vi "Bernards_2_2400.vi"() -> ()   [LabVIEW 2018]
uses:
  <vilib>/Utility/file.llb/Write Delimited Spreadsheet (string).vi
  <instrlib>/Keithley 24XX/Public/Data/Read (Single Point).vi
  <instrlib>/Keithley 24XX/Keithley 24XX.lvlib
  <vilib>/Analysis/NI_AALBase.lvlib
panel:
  out "Current (A) 2":dbl format="%.2e"
  out "error 8":string
  in  "Keithley 2401 (new)\nVISA resource #2 = 22":refnum<visa-resource-name>="GPIB0::22::INSTR"
  in  "Delay Gate (s) 2":dbl=60.0 format="%#.3g"
  in  "source/measure (V/I:0)":u16(ring)=1 items=["voltage/current", "current/voltage"]
  in  "Setpoint Array":dbl[](array[numeric])=[-2e-08, -5e-08, -1e-07]
  in  "Measurement Speed (1 PLC)":dbl=1.0 format="%.2g"
  in  "Initial Gate Setting":dbl format="%#.3e"
  in  "Voltage Compliance Limit 2401 (V)":dbl=-0.95 format="%#.3f"
  in  "Current Compliance\nLimit 2401 (A)":dbl=0.10000000009313226
  in  "Delay Gate (s)":dbl=30.0 format="%#.3g"
  in  "Keithley 237 GPIB address":string="17"
  in  "Wait Time Btwn Keithley Readings (ms)":i32=30
  out "Time Btwn Iterations (ms)":i32
  out "Total Elapsed Time (ms)":i32
  out "# Avgs":i32
  out "Current (A)":dbl format="%.2e"
  in  "Total Measure Time (s)":dbl=120.0 format="%#.3g"
  in  "Drain Bias (V)":dbl=-0.6 format="%#.3g"
  in  "Current Compliance\nLimit (A)":dbl=0.5 format="%#.3e"
  in  "Keithley 2400 (old)\nVISA resource #1 = 24":refnum<visa-resource-name>="GPIB0::24::INSTR"
  in  "ApproximateTime Step (ms)":dbl=300.0 format="%#.3g"
  in  "Current Offset":dbl format="%^#_3e"
  out "I-t Measurement\nBy M. Ziffer 7/3/2014":cluster{dbl[], dbl[]}(graph)={[-2.0, -1.95, -1.9, -1.85, -1.8, -1.75, -1.7, -1.65, -1.6, -1.55, -1.5, -1.45, -1.4, -1.35, -1.2999999999999998, -1.25, -1.2, -1.15, -1.1, -1.0499999999999998, -1.0, -0.95, -0.8999999999999999, -0.8499999999999999, -0.7999999999999998, -0.75, -0.7, -0.6499999999999999, -0.5999999999999999, -0.5499999999999998, -0.5, -0.44999999999999996, -0.3999999999999999, -0.34999999999999987, -0.2999999999999998, -0.25, -0.19999999999999996, -0.1499999999999999, -0.09999999999999987, -0.04999999999999982, 0.0, 0.050000000000000266, 0.10000000000000009, 0.1499999999999999, 0.20000000000000018, 0.25, 0.30000000000000027, 0.3500000000000001, 0.40000000000000036, 0.4500000000000002, 0.5, 0.5500000000000003, 0.6000000000000001, 0.6500000000000004, 0.7000000000000002, 0.75, 0.8000000000000003, 0.8500000000000001, 0.9000000000000004, 0.9500000000000002, 1.0, 1.0500000000000003, 1.1, 1.1500000000000004, 1.2000000000000002, 1.25, 1.3000000000000003, 1.35, 1.4000000000000004, 1.4500000000000002, 1.5, 1.5500000000000003, 1.6, 1.6500000000000004, 1.7000000000000002, 1.75, 1.8000000000000003, 1.85, 1.9000000000000004, 1.9500000000000002, 2.0, 1.95, 1.9, 1.85, 1.8, 1.75, 1.7, 1.65, 1.6, 1.55, 1.5, 1.45, 1.4, 1.35, 1.2999999999999998, 1.25, 1.2, 1.15, 1.1, 1.0499999999999998, 1.0, 0.95, 0.8999999999999999, 0.8499999999999999, 0.7999999999999998, 0.75, 0.7, 0.6499999999999999, 0.5999999999999999, 0.5499999999999998, 0.5, 0.44999999999999996, 0.3999999999999999, 0.34999999999999987, 0.2999999999999998, 0.25, 0.19999999999999996, 0.1499999999999999, 0.09999999999999987, 0.04999999999999982, 0.0, -0.050000000000000266, -0.10000000000000009, -0.1499999999999999, -0.20000000000000018, -0.25, -0.30000000000000027, -0.3500000000000001, -0.40000000000000036, -0.4500000000000002, -0.5, -0.5500000000000003, -0.6000000000000001, -0.6500000000000004, -0.7000000000000002, -0.75, -0.8000000000000003, -0.8500000000000001, -0.9000000000000004, -0.9500000000000002, -1.0, -1.0500000000000003, -1.1, -1.1500000000000004, -1.2000000000000002, -1.25, -1.3000000000000003, -1.35, -1.4000000000000004, -1.4500000000000002, -1.5, -1.5500000000000003, -1.6, -1.6500000000000004, -1.7000000000000002, -1.75, -1.8000000000000003, -1.85, -1.9000000000000004, -1.9500000000000002, -2.0], [-0.9617289445307117, -0.9618513744908972, -0.9601574911889584, -0.9603488957746004, -0.9598860982876659, -0.9595594700613103, -0.9590290885663679, -0.9586886097902229, -0.9580144940757807, -0.9570474587019399, -0.9571418538143588, -0.9562287187728303, -0.9551771894828052, -0.9535572870291384, -0.9535421571112963, -0.9533114258642045, -0.9520938012261039, -0.9513117179729429, -0.9508812384355169, -0.9504840780921618, -0.9504173840793213, -0.9482281628421478, -0.9464640811713977, -0.9453356785488072, -0.9439408336230415, -0.9428695575652444, -0.9416178906119992, -0.9396031084275935, -0.9378375248899987, -0.9354517815949719, -0.9324159524550173, -0.928767917889437, -0.9245502864168607, -0.9203528467096396, -0.9146985405384399, -0.908595454304189, -0.9012966039381313, -0.8917361646028689, -0.8808115851751085, -0.8684870433493713, -0.853007079283089, -0.8360736418594031, -0.8154860511533626, -0.7920970894092216, -0.7641180332150388, -0.7294003786125389, -0.6854183749419586, -0.6263231964633708, -0.5399961516707377, -0.4044042921440459, -0.19129744134883978, 0.11936942255465804, 0.5420583260977958, 1.0996962734707192, 1.8318907919106253, 2.7834859177196174, 3.9948214605959804, 5.494887344369723, 7.293988211209965, 9.39251059714275, 11.765998658717283, 14.371720946722268, 17.153138293174568, 20.070768287470067, 23.082285540692517, 26.15604905590766, 29.26009131920428, 32.38734131897913, 35.54092126952808, 38.70923397757575, 41.89103456238207, 45.09512285116253, 48.318234786641504, 51.57411300669423, 54.84161623237131, 58.130390342544004, 61.4596508891188, 64.79419021952893, 68.17503711098149, 71.57587551887687, 75.0023346626475, 71.8977923333163, 68.72637799211101, 65.51757272894447, 62.2950059155054, 59.076872390492845, 55.84672949319313, 52.615591470047114, 49.383497814590335, 46.15858586388574, 42.93308596012382, 39.714879010509975, 36.494540522470736, 33.276879251143754, 30.087779593472593, 26.903443634933772, 23.758388169345494, 20.669969771208738, 17.671195580039395, 14.804861569698371, 12.12778391916459, 9.68736655227705, 7.528128139792144, 5.673530623057721, 4.128839936603901, 2.8787577310032053, 1.895544581260216, 1.1383875896205915, 0.5622048852612092, 0.12746496878202787, -0.18928305409978952, -0.4042961076690051, -0.5411369085387429, -0.6286316214282486, -0.6871327837574404, -0.7298882072135505, -0.7640718647157413, -0.7921132761963248, -0.8155779431543743, -0.8358809022810104, -0.8523300154596555, -0.8668520109778625, -0.8802307520791266, -0.8907705198464766, -0.8998007445608903, -0.9078572589377096, -0.9150023626386364, -0.9215738644543149, -0.925261336930741, -0.9288795566582202, -0.9332418679701618, -0.9352489739462505, -0.9376688708058178, -0.9394550911063516, -0.9405290371496502, -0.9430050037047499, -0.9440335043698243, -0.9453382929096107, -0.9473152502994113, -0.9474565926568992, -0.9494901203645137, -0.94896546821346, -0.9503187058651598, -0.9511280452203158, -0.9523093469306558, -0.9532668704811476, -0.9541692143312739, -0.9545545822386634, -0.955485183435348, -0.9561708134622656, -0.956805602515258, -0.9577699122788996, -0.9578049002139094, -0.9580356870856992, -0.958780001168953, -0.9592832934359943, -0.9588639388381576, -0.959203916992021, -0.9603773199952523, -0.9611007191920772, -0.9623172869609168]}
  in  "First bias settle (ms)":dbl=2000.0 format="%#.2f"
  out "Outputfile":path
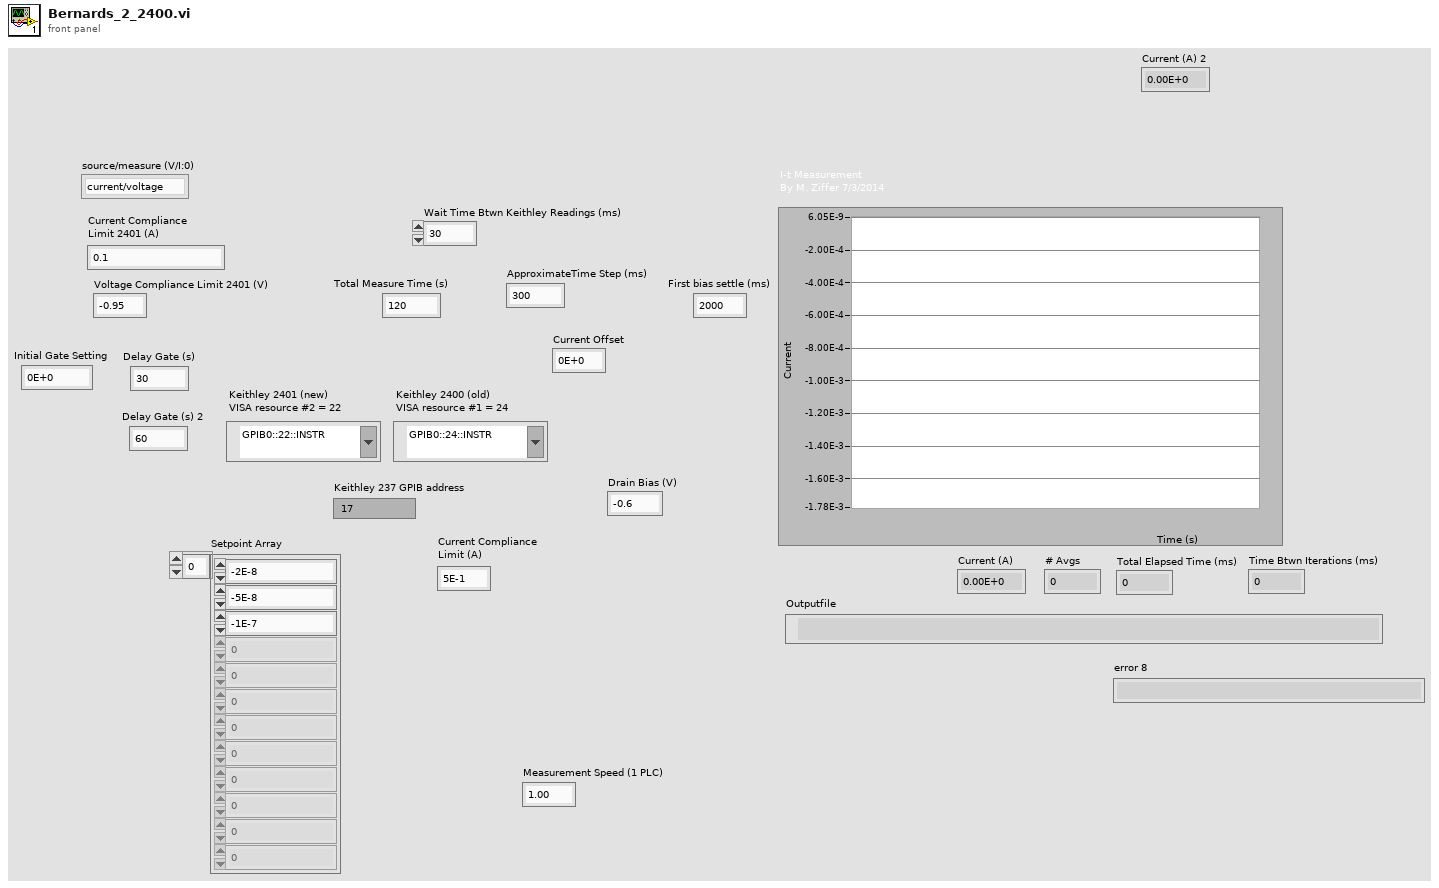
[diagram p1: front panel]
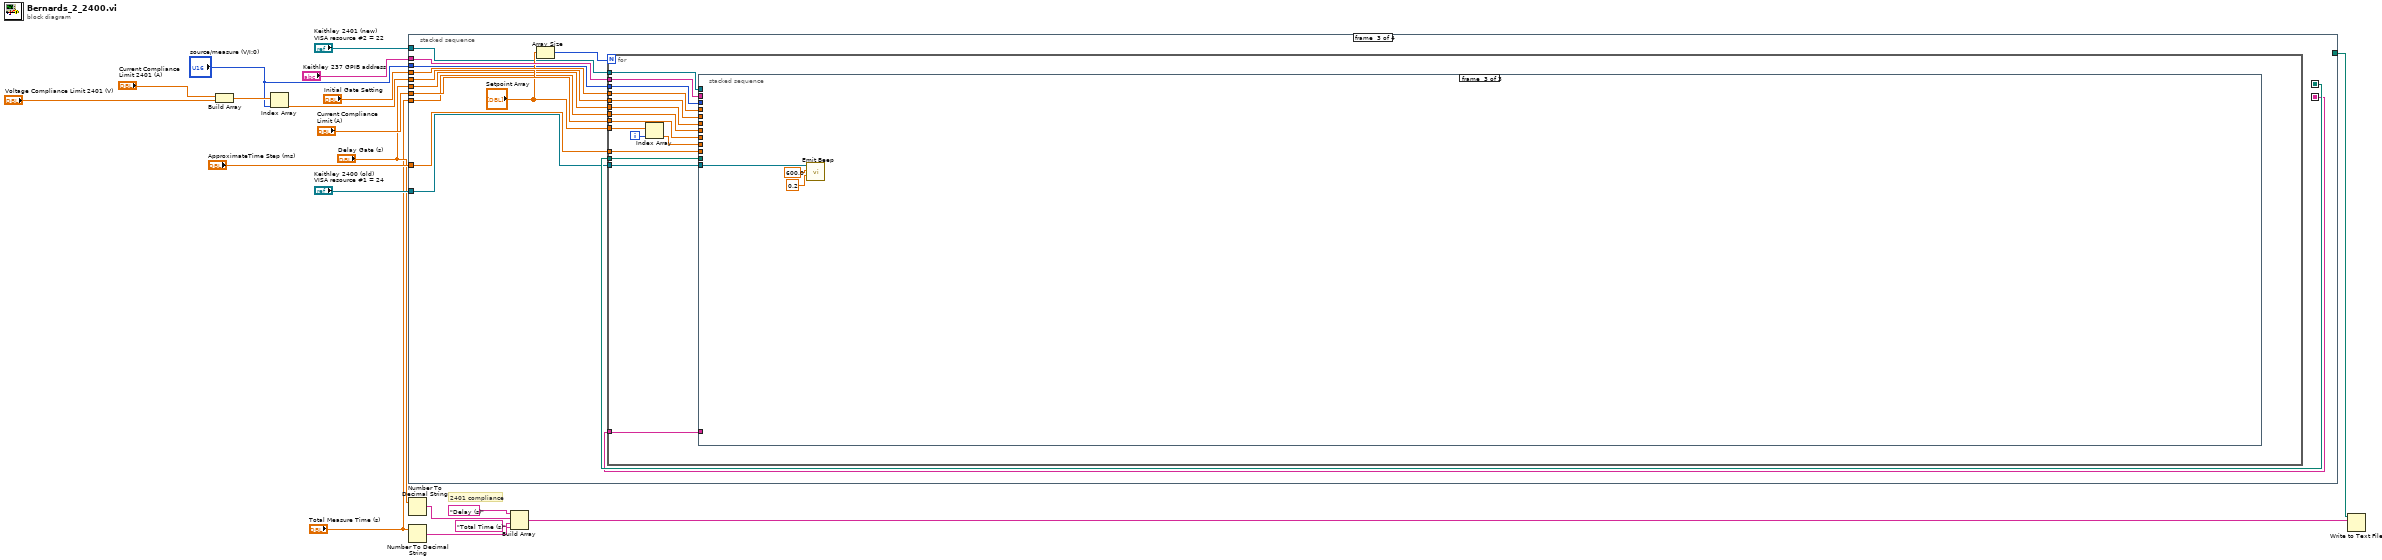
[diagram p0: block diagram]
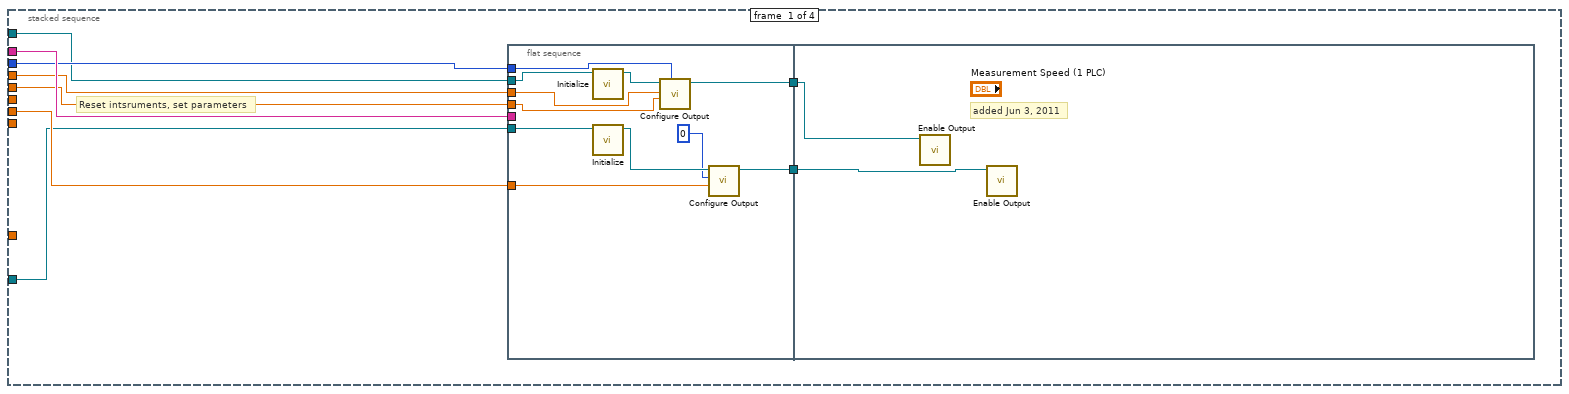
[diagram p2: hidden frame]
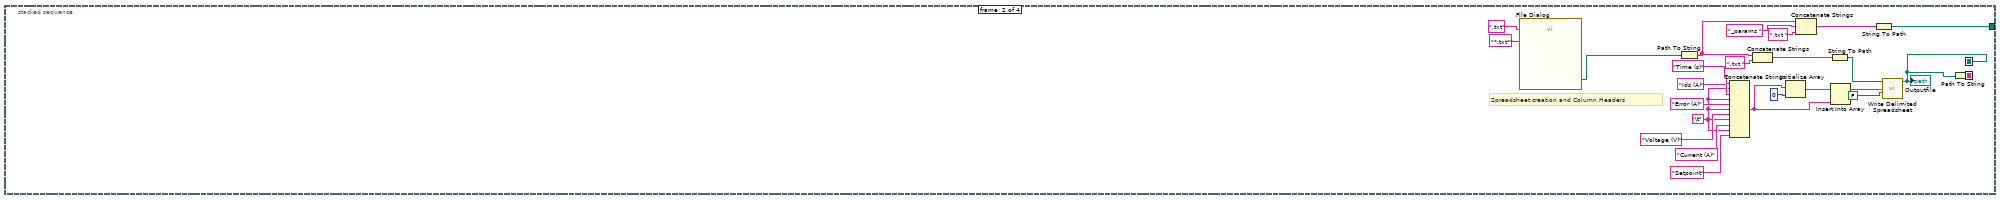
[diagram p3: hidden frame]
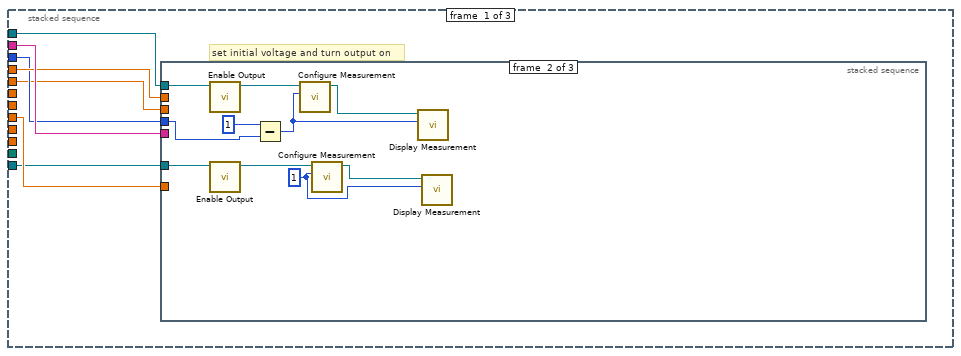
[diagram p4: hidden frame]
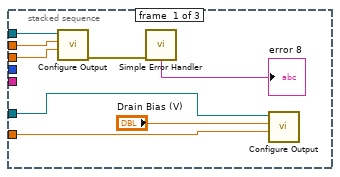
[diagram p5: hidden frame]
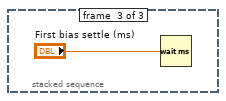
[diagram p6: hidden frame]
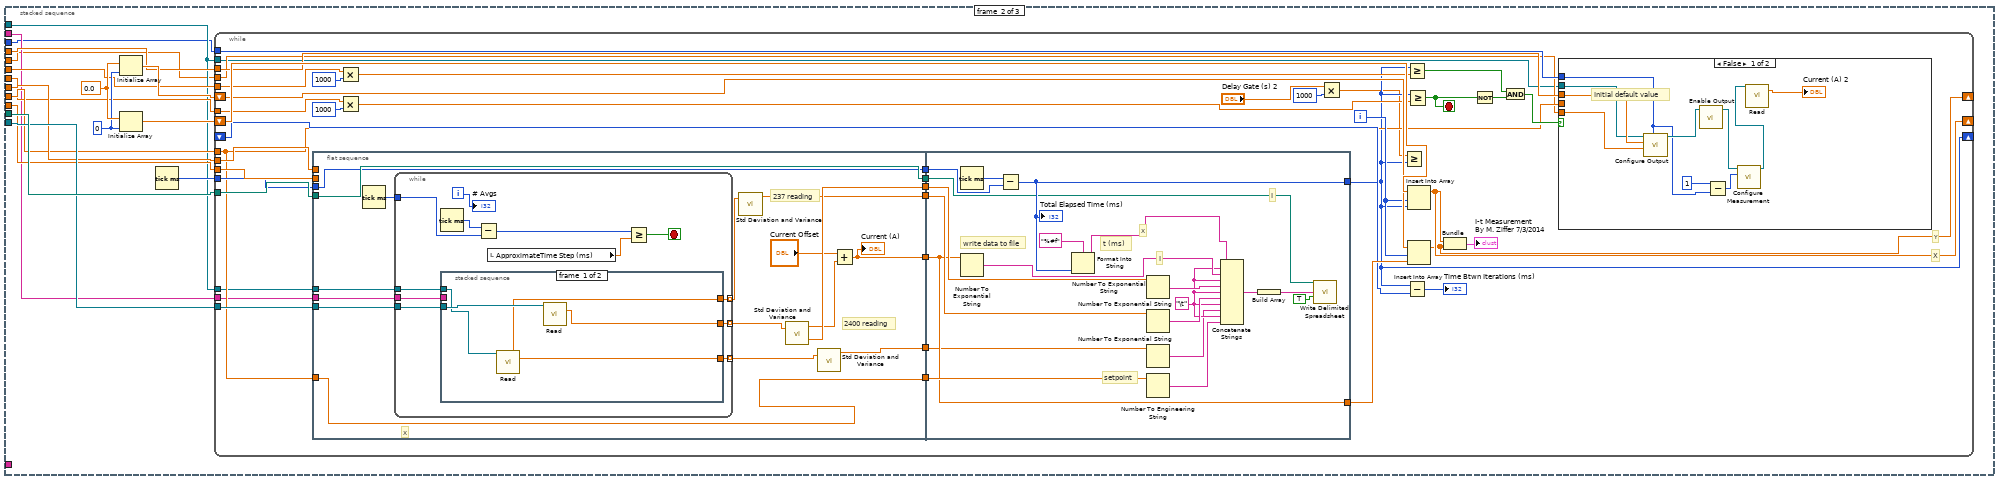
[diagram p7: hidden frame]
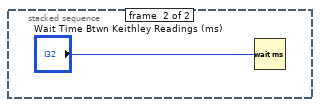
[diagram p8: hidden frame]
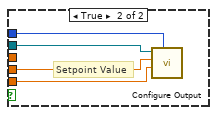
[diagram p9: hidden frame]
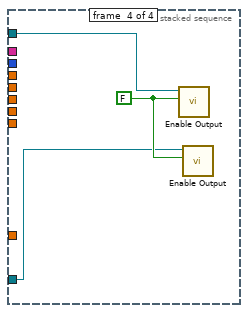
[diagram p10: hidden frame]
diagram:
  # "2401 compliance"
  n1 = Build Array("Current Compliance\nLimit 2401 (A)", "Voltage Compliance Limit 2401 (V)") -> (w4:dbl[])
  n2 = Index Array(array=w4, index="source/measure (V/I:0)") -> (element=w2:dbl)
  n3 = stacked-sequence {
    seq-local: [_ w47 _ _] -> [_ _ w79 _]
    seq-local: [_ w66 _ _] -> [_ _ w78 _]
    tunnel: "ApproximateTime Step (ms)" -> [_ _ w80 _]
    tunnel: "Keithley 2400 (old)\nVISA resource #1 = 24" -> [w27 _ w76 w252]
    tunnel: "Current Compliance\nLimit (A)" -> [w28 _ w77 _]
    tunnel: "Keithley 237 GPIB address" -> [w26 _ w74 _]
    tunnel: "Initial Gate Setting" -> [w22 _ w75 _]
    tunnel: "source/measure (V/I:0)" -> [w25 _ w68 _]
    tunnel: [_ w42 _ _] -> w13
    tunnel: "Delay Gate (s)" -> [_ _ w71 _]
    tunnel: "Total Measure Time (s)" -> [_ _ w70 _]
    tunnel: "Keithley 2401 (new)\nVISA resource #2 = 22" -> [w24 _ w69 w253]
    tunnel: w2 -> [w23 _ w67 _]
    frame #0 {
      # "Reset intsruments, set parameters"
      n4 = flat-sequence {
        tunnel: w27 -> [w38]
        tunnel: w28 -> [w34]
        tunnel: w26 -> [_]
        tunnel: w25 -> [w33]
        tunnel: w24 -> [w36]
        tunnel: w23 -> [w32]
        tunnel: w22 -> [w31]
        tunnel: [w39] -> w21
        tunnel: [w29] -> w20
        tunnel: w21 -> [w41]
        tunnel: w20 -> [w40]
        frame #0 {
          n5 = call <instrlib>:"Initialize.vi"("VISA resource name"=w36) -> ("VISA resource name out"=w35:refnum<visa-resource-name>)  [unwired: 9 in, 1 out]
          n6 = call <instrlib>:"Initialize.vi"("VISA resource name"=w38) -> ("VISA resource name out"=w37:refnum<visa-resource-name>)  [unwired: 9 in, 1 out]
          n7 = call <instrlib>:"Configure Output.vi"("Source Mode  (0: Voltage)"=w33, "Compliance  Level (0.1)"=w32, "Output Level (0)"=w31, "VISA resource name"=w35) -> ("VISA resource name out"=w29:refnum<visa-resource-name>)  [unwired: 2 in, 5 out]
          n8 = call <instrlib>:"Configure Output.vi"("Compliance  Level (0.1)"=w34, "Output Level (0)"=0, "VISA resource name"=w37) -> ("VISA resource name out"=w39:refnum<visa-resource-name>)  [unwired: 3 in, 5 out]
        }
        frame #1 {
          # "added Jun 3, 2011"
          n9 = call <instrlib>:"Enable Output.vi"("VISA resource name"=w40) -> ()  [unwired: 2 in, 9 out]
          n10 = call <instrlib>:"Enable Output.vi"("VISA resource name"=w41) -> ()  [unwired: 2 in, 9 out]
        }
      }
    }
    frame #1 {
      w49 = "\t"
      # "Spreadsheet creation and Column Headers"
      n11 = call "File Dialog"("default name"=".txt", "pattern (all files)"="*.txt*") -> ("selected path"=w53:path)  [unwired: 5 in, 8 out]
      n12 = Path To String(path=w53) -> (string=w44:string)
      n13 = Concatenate Strings("Time (s)", w49, "Ids (A)", w49, "Error (A)", w49, "Voltage (V)", w49, "Current (A)", w49, "Setpoint") -> (w64:string)
      n14 = Concatenate Strings(w44, ".txt " ("string")) -> (w52:string)
      n15 = Initialize Array(w64, 0 ("dimension size")) -> (w63:string[])
      n16 = Concatenate Strings(w44, "_params " ("string"), ".txt " ("string")) -> (w43:string)
      n17 = String To Path(string=w52) -> (path=w51:path)
      n18 = Insert Into Array(array=w63, new element=w64) -> (w56:string[])  [unwired: 1 in]
      n19 = String To Path(string=w43) -> (path=w42:path)
      n20 = call-poly <vilib>:"Write Delimited Spreadsheet.vi"("file path (dialog if empty)"=w51, "1D data"=w56, "append to file? (new file:F)"=FALSE) -> ("new file path (Not A Path if cancelled)"=w47:path)  [unwired: 11 in, 1 out]
      "Outputfile" <- w47
      n21 = Path To String(path=w47) -> (string=w66:string)
    }
    frame #2 {
      n22 = Array Size(array="Setpoint Array") -> (size(s)=w72:i32)
      n23 = for {
        N: w72 -> [_]
        tunnel: w80 -> [w95]
        tunnel: w79 -> [w94]
        tunnel: w78 -> [w93]
        tunnel: w77 -> [w92]
        tunnel: w76 -> [w91]
        tunnel: w75 -> [w90]
        tunnel: w74 -> [w84]
        tunnel: "Setpoint Array" -> [w89]
        tunnel: w71 -> [w86]
        tunnel: w70 -> [w85]
        tunnel: w69 -> [w83]
        tunnel: w68 -> [w82]
        tunnel: w67 -> [w81]
        i -> [w87]
        n24 = Index Array(array=w89, index=w87) -> (element=w88:dbl)
        n25 = stacked-sequence {
          tunnel: w95 -> [_ w131 _]
          tunnel: w94 -> [_ w138 _]
          tunnel: w93 -> [_ _ _]
          tunnel: w92 -> [w102 w132 _]
          tunnel: w91 -> [w101 w133 w251]
          tunnel: w90 -> [w98 w129 _]
          tunnel: w84 -> [w100 w125 _]
          tunnel: w88 -> [_ w128 _]
          tunnel: w86 -> [_ w127 _]
          tunnel: w85 -> [_ w126 _]
          tunnel: w83 -> [w99 w124 _]
          tunnel: w82 -> [w97 w123 _]
          tunnel: w81 -> [w96 w122 _]
          frame #0 {
            # "set initial voltage and turn output on"
            n26 = stacked-sequence {
              tunnel: w101 -> [w109 w120 _]
              tunnel: w102 -> [w110 _ _]
              tunnel: w100 -> [_ _ _]
              tunnel: w99 -> [w107 w119 _]
              tunnel: w98 -> [w106 _ _]
              tunnel: w97 -> [_ w115 _]
              tunnel: w96 -> [w105 _ _]
              frame #0 {
                n27 = call <instrlib>:"Configure Output.vi"("Compliance  Level (0.1)"=w105, "Output Level (0)"=w106, "VISA resource name"=w107) -> ("error out"=w104:errorcluster)  [unwired: 3 in, 5 out]
                n28 = call <vilib>:"Simple Error Handler.vi"("error in (no error)"=w104) -> ("message"=→"error 8":string)  [unwired: 1 in, 7 out]
                n29 = call <instrlib>:"Configure Output.vi"("Compliance  Level (0.1)"=w110, "Output Level (0)"="Drain Bias (V)", "VISA resource name"=w109) -> ()  [unwired: 3 in, 6 out]
              }
              frame #1 {
                w111 = 1
                n30 = call <instrlib>:"Enable Output.vi"("VISA resource name"=w119) -> ("VISA resource name out"=w118:refnum<visa-resource-name>)  [unwired: 2 in, 8 out]
                n31 = call <instrlib>:"Enable Output.vi"("VISA resource name"=w120) -> ("VISA resource name out"=w117:refnum<visa-resource-name>)  [unwired: 2 in, 8 out]
                n32 = Subtract(x=1, y=w115) -> (x-y=w112:i32)
                n33 = call <instrlib>:"Configure Measurement.vi"("Function (0: Volts)"=w112, "VISA resource name"=w118) -> ("VISA resource name out"=w113:refnum<visa-resource-name>)  [unwired: 8 in, 1 out]
                n34 = call <instrlib>:"Configure Measurement.vi"("Function (0: Volts)"=w111, "VISA resource name"=w117) -> ("VISA resource name out"=w114:refnum<visa-resource-name>)  [unwired: 8 in, 1 out]
                n35 = call <instrlib>:"Display Measurement.vi"("Displayed Measurement (0: Voltage)"=w112, "VISA resource name"=w113) -> ()  [unwired: 8 in, 2 out]
                n36 = call <instrlib>:"Display Measurement.vi"("Displayed Measurement (0: Voltage)"=w111, "VISA resource name"=w114) -> ()  [unwired: 8 in, 2 out]
              }
              frame #2 {
                n37 = Wait (ms)(milliseconds to wait="First bias settle (ms)") -> ()  [unwired: 1 out]
              }
            }
          }
          frame #1 {
            w134 = 0
            w135 = 0.0
            n38 = Initialize Array(w135, w134) -> (w136:dbl[])
            n39 = Initialize Array(w135, w134) -> (w137:dbl[])
            n40 = Tick Count (ms)() -> (millisecond timer value=w130:u32)
            n41 = while {
              shift-left: w136 -> [w177]
              shift-right: [w172] -> _
              shift-left: w137 -> [w178]
              shift-right: [w174] -> _
              tunnel: w138 -> [w179]
              tunnel: w133 -> [w176]
              tunnel: w132 -> [w175]
              tunnel: w131 -> [w170]
              tunnel: w130 -> [w165]
              shift-right: [w147] -> _
              shift-left: _ -> [w169]
              tunnel: w125 -> [w156]
              tunnel: w129 -> [w162]
              tunnel: w128 -> [w157]
              tunnel: w127 -> [w144]
              tunnel: w126 -> [w143]
              tunnel: w124 -> [w142]
              tunnel: w124 -> [w139]
              tunnel: w123 -> [w141]
              tunnel: w122 -> [w140]
              i -> [w171]
              stop <- w161 stop-if-true
              # "X"
              # "X"
              # "Y"
              n42 = flat-sequence {
                tunnel: w179 -> [w190]
                tunnel: [w190] -> w155
                tunnel: w176 -> [w184]
                tunnel: w175 -> [_]
                tunnel: w170 -> [_]
                tunnel: w165 -> [w189]
                tunnel: [w189] -> w154
                tunnel: w157 -> [w188]
                tunnel: [w188] -> w153
                tunnel: w156 -> [w191]
                tunnel: [w196] -> w152
                tunnel: [w192] -> w151
                tunnel: [w187] -> w150
                tunnel: [w186] -> w145
                tunnel: w142 -> [w185]
                tunnel: [w220] -> w173
                tunnel: w155 -> [w215]
                tunnel: w154 -> [w227]
                tunnel: [w226] -> w147
                tunnel: w153 -> [w223]
                tunnel: w152 -> [w229]
                tunnel: w151 -> [w220]
                tunnel: w150 -> [w222]
                tunnel: w145 -> [w216]
                frame #0 {
                  # "2400 reading"
                  # "237 reading"
                  n43 = Tick Count (ms)() -> (millisecond timer value=w193:u32)
                  n44 = while {
                    tunnel: w193 -> [w207]
                    tunnel: w191 -> [w202]
                    tunnel: w185 -> [w201]
                    tunnel: w184 -> [w200]
                    tunnel: [w199] -> w183 mode=indexing
                    tunnel: [w198] -> w182 mode=indexing
                    tunnel: [w197] -> w181 mode=indexing
                    i -> [w208]
                    stop <- w205 stop-if-true
                    n45 = Tick Count (ms)() -> (millisecond timer value=w204:u32)
                    n46 = stacked-sequence {
                      tunnel: w202 -> [_ _]
                      tunnel: w201 -> [w212 _]
                      tunnel: w200 -> [w213 _]
                      tunnel: [w211 _] -> w199
                      tunnel: [w210 _] -> w198
                      tunnel: [w209 _] -> w197
                      frame #0 {
                        n47 = call-poly <instrlib>:"Read.vi"("VISA resource name"=w212) -> ("Voltage"=w210:sgl, "Current"=w209:sgl)  [unwired: 8 in, 5 out]
                        n48 = call-poly <instrlib>:"Read.vi"("VISA resource name"=w213) -> ("Current"=w211:sgl)  [unwired: 8 in, 6 out]
                      }
                      frame #1 {
                        n49 = Wait (ms)(milliseconds to wait="Wait Time Btwn Keithley Readings (ms)") -> ()  [unwired: 1 out]
                      }
                    }
                    n50 = Subtract(x=w204, y=w207) -> (x-y=w206:u32)
                    n51 = local read "ApproximateTime Step (ms)"() -> (w203:dbl)
                    n52 = Greater Or Equal?(x=w206, y=w203) -> (x >= y?=w205:bool)
                    "# Avgs" <- w208
                  }
                  n53 = call <vilib>:"Std Deviation and Variance.vi"("X"=w182) -> ("mean"=w187:dbl)  [unwired: 1 in, 2 out]
                  n54 = call <vilib>:"Std Deviation and Variance.vi"("X"=w183) -> ("mean"=w195:dbl, "standard deviation"=w196:dbl)  [unwired: 1 in, 1 out]
                  n55 = call <vilib>:"Std Deviation and Variance.vi"("X"=w181) -> ("mean"=w186:dbl)  [unwired: 1 in, 2 out]
                  n56 = Add(x="Current Offset", y=w195) -> (x+y=w192:dbl)
                  "Current (A)" <- w192
                }
                frame #1 {
                  w218 = "\t"
                  # "setpoint"
                  # "I"
                  # "I"
                  # "t (ms)"
                  # "write data to file"
                  # "X"
                  n57 = Tick Count (ms)() -> (millisecond timer value=w228:u32)
                  n58 = Number To Exponential String(number=w220) -> (E-format string=w232:string)  [unwired: 3 out]
                  n59 = Subtract(x=w228, y=w227) -> (x-y=w226:u32)
                  "Total Elapsed Time (ms)" <- w226
                  n60 = Format Into String(format string="%#f", w226) -> (resulting string=w233:string)  [unwired: 2 in, 1 out]
                  n61 = Number To Exponential String(number=w229) -> (E-format string=w230:string)  [unwired: 3 out]
                  n62 = Number To Exponential String(number=w222) -> (E-format string=w221:string)  [unwired: 3 out]
                  n63 = Number To Exponential String(number=w216) -> (E-format string=w217:string)  [unwired: 3 out]
                  n64 = Number To Engineering String(4:w223) -> (0:w219:string)  [unwired: 3 in]
                  n65 = Concatenate Strings(w233, w218, w232, w218, w230, w218, w221, w218, w217, w218, w219) -> (w231:string)
                  n66 = Build Array(w231) -> (w225:string[])
                  n67 = call-poly <vilib>:"Write Delimited Spreadsheet.vi"("file path (dialog if empty)"=w215, "1D data"=w225, "append to file? (new file:F)"=TRUE) -> ()  [unwired: 11 in, 2 out]
                }
              }
              n68 = Multiply(x=w144, y=1000) -> (x*y=w164:dbl)
              n69 = Multiply(x=w143, y=1000) -> (x*y=w166:dbl)
              n70 = Multiply(x="Delay Gate (s) 2", y=1000) -> (x*y=w146:dbl)
              n71 = Greater Or Equal?(x=w146, y=w147) -> ()  [unwired: 1 out]
              n72 = Greater Or Equal?(x=w147, y=w164) -> (x >= y?=w159:bool)
              n73 = Subtract(x=w147, y=w169) -> (x-y=→"Time Btwn Iterations (ms)":u32)
              n74 = Greater Or Equal?(x=w147, y=w166) -> (x >= y?=w161:bool)
              n75 = Insert Into Array(array=w178, index=w171, new element=w147) -> (w174:dbl[])
              n76 = Insert Into Array(array=w177, index=w171, new element=w173) -> (w172:dbl[])
              n77 = Bundle(w174, w172) -> (→"I-t Measurement\nBy M. Ziffer 7/3/2014":cluster{dbl[], dbl[]})  [unwired: 1 out]
              n78 = Not(x=w161) -> (.not. x?=w160:bool)
              n79 = And(x=w159, y=w160) -> (x .and. y?=w158:bool)
              n80 = case shown="False" w158 {
                tunnel: w162 -> [w244 _]
                tunnel: w157 -> [_ w248]
                tunnel: w139 -> [w243 w247]
                tunnel: w141 -> [w236 w246]
                tunnel: w140 -> [w242 w245]
                frame False {
                  # "Initial default value"
                  n81 = call <instrlib>:"Configure Output.vi"("Source Mode  (0: Voltage)"=w236, "Compliance  Level (0.1)"=w242, "Output Level (0)"=w244, "VISA resource name"=w243) -> ("VISA resource name out"=w239:refnum<visa-resource-name>)  [unwired: 2 in, 5 out]
                  n82 = call <instrlib>:"Enable Output.vi"("VISA resource name"=w239) -> ("VISA resource name out"=w238:refnum<visa-resource-name>)  [unwired: 9 in, 1 out]
                  n83 = Subtract(x=1, y=w236) -> (x-y=w235:i32)
                  n84 = call <instrlib>:"Configure Measurement.vi"("Function (0: Volts)"=w235, "VISA resource name"=w238) -> ("VISA resource name out"=w237:refnum<visa-resource-name>)  [unwired: 8 in, 1 out]
                  n85 = call-poly <instrlib>:"Read.vi"("VISA resource name"=w237) -> ("Voltage"=→"Current (A) 2":sgl)  [unwired: 8 in, 6 out]
                }
                frame True {
                  # "Setpoint Value"
                  n86 = call <instrlib>:"Configure Output.vi"("Source Mode  (0: Voltage)"=w246, "Compliance  Level (0.1)"=w245, "Output Level (0)"=w248, "VISA resource name"=w247) -> ()  [unwired: 2 in, 6 out]
                }
              }
            }
          }
          frame #2 {
            n87 = call <instrlib>:"Emit Beep.vi"("Beep Duration (.25 s)"=0.2, "Beep Frequency (300)"=600.0, "VISA resource name"=w251) -> ()  [unwired: 7 in, 2 out]
          }
        }
      }
    }
    frame #3 {
      w254 = FALSE
      n88 = call <instrlib>:"Enable Output.vi"("Enable Output (T: Enable)"=w254, "VISA resource name"=w253) -> ()  [unwired: 8 in, 2 out]
      n89 = call <instrlib>:"Enable Output.vi"("Enable Output (T: Enable)"=w254, "VISA resource name"=w252) -> ()  [unwired: 8 in, 2 out]
    }
  }
  n90 = Number To Decimal String(number="Delay Gate (s)") -> (decimal integer string=w12:string)  [unwired: 1 in]
  n91 = Number To Decimal String(number="Total Measure Time (s)") -> (decimal integer string=w9:string)  [unwired: 1 in]
  n92 = Build Array("Delay (s)", w12, "Total Time (s)", w9) -> (w15:string[])
  n93 = Write to Text File(file (use dialog)=w13, text=w15) -> ()  [unwired: 2 in, 3 out]
